vi "Main.vi"(8 "error in (no error)":errorcluster, 11 "Dispatcher in":refnum<class "Dispatcher Thread.lvclass">) -> (0 "error out":errorcluster, 3 "Dispatcher out":refnum<class "Dispatcher Thread.lvclass">)   [LabVIEW 2019, in "DSF Core.lvlib" / "Dispatcher Thread.lvclass"]
uses:
  Dispatcher Thread.lvclass
  C:/Dev/GitHub/niveristand-data-sharing-framework-custom-device/Core/Classes/Thread/Thread.lvclass
  Interface/Dispatcher/Command.ctl
  Thread.lvclass
  Interface/Dispatcher/Dispatcher Interface.lvclass
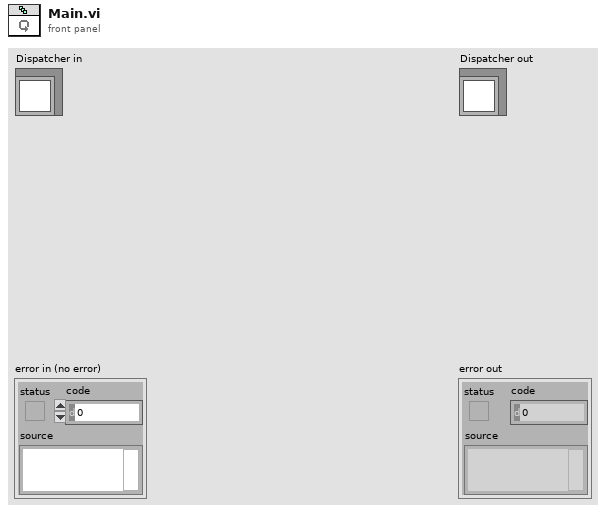
[diagram p1: front panel]
types:
  T1 = typedef "DSF Core.lvlib/Dispatcher Interface.lvclass/Command.ctl" = enum8{"Idle", "Start", "Rx", "Tx", "Set Inline Buffer", "Shutdown", "Error"}
  T2 = typedef "DSF Core.lvlib/Dispatcher Interface.lvclass/Command Data.ctl" = cluster{"Command":T1, "Parameters":T3}
  T3 = typedef "DSF Core.lvlib/Dispatcher Interface.lvclass/Parameters.ctl" = cluster{"arg1":u64, "arg2":u64}
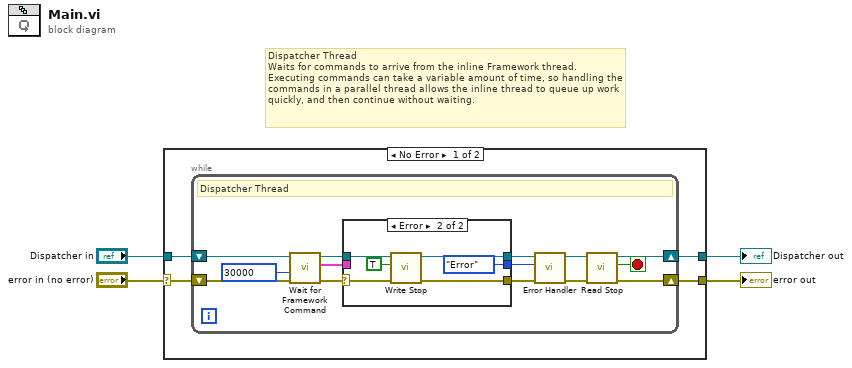
[diagram p0: block diagram]
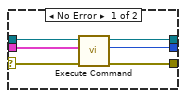
[diagram p2: hidden frame]
diagram:
  # "Dispatcher Thread\nWaits for commands to arrive from the inline Framework thread. Executing commands can take a variable amount of time, so handling the commands in a parallel thread allows the inline thread to queue up work quickly, and then continue without waiting."
  n1 = case shown="No Error" "error in (no error)" {
    selector: "error in (no error)" -> [w5 w36]
    tunnel: [w8 w36] -> w4
    tunnel: [w7 w35] -> w3
    tunnel: "Dispatcher in" -> [w6 w35]
    frame No Error {
      n2 = while {
        shift-right: [w18] -> w8
        shift-left: w5 -> [w15]
        shift-right: [w10] -> w7
        shift-left: w6 -> [w11]
        stop <- w17 stop-if-true
        # "Dispatcher Thread"
        n3 = call "Wait for Framework Command.vi"("error in (no error)"=w15, "timeout in ms (5000)"=30000 ("timeout in ms (0)"), "Dispatcher in"=w11) -> ("error out"=w13:errorcluster, "command"=w12:T2, "Dispatcher out"=w14:refnum<class "Dispatcher Thread.lvclass">)  [unwired: 6 in]
        n4 = case shown="Error" w13 {
          selector: w13 -> [w23 w31]
          tunnel: [w26 w29] -> w22
          tunnel: [w28 w30] -> w21
          tunnel: w14 -> [w27 w32]
          tunnel: w12 -> [w24 _]
          tunnel: [w25 Command."Error" ("state")] -> w9
          frame No Error {
            n5 = call "Execute Command.vi"("error in (no error)"=w23, "command"=w24, "Dispatcher in"=w27) -> ("error out"=w28:errorcluster, "state"=w25:T1, "Dispatcher out"=w26:refnum<class "Dispatcher Thread.lvclass">)  [unwired: 6 in]
          }
          frame Error {
            n6 = call "Write Stop.vi"("error in (no error)"=w31, "stop"=TRUE, "Thread in"=w32) -> ("error out"=w30:errorcluster, "Thread out"=w29:refnum<class "Dispatcher Thread.lvclass">)  [unwired: 7 in]
          }
        }
        n7 = call "Error Handler.vi"("error in"=w21, "state"=w9, "dispatcher in"=w22) -> ("error out"=w19:errorcluster, "dispatcher out"=w20:refnum<class "Dispatcher Thread.lvclass">)  [unwired: 7 in]
        n8 = call "Read Stop.vi"("error in (no error)"=w19, "Thread in"=w20) -> ("error out"=w18:errorcluster, "stop"=w17:bool, "Thread out"=w10:refnum<class "Dispatcher Thread.lvclass">)  [unwired: 7 in]
      }
    }
    frame Error {
    }
  }
  "error out" <- w4
  "Dispatcher out" <- w3
